vi "Read Configured Load DeviceIDs.vi"(8 "error in":errorcluster, 11 "EMS Generic in":refnum<class "EMS Generic.lvclass">) -> (0 "error out":errorcluster, 2 "Load DeviceIDs":T1[](array[typedef]), 3 "EMS Generic out":refnum<class "EMS Generic.lvclass">)   [LabVIEW 2018, in "EMS Generic Actor.lvlib" / "EMS Generic.lvclass"]
uses:
  EMS Generic.lvclass
  <vilib>/ORNL/CSEISMIC DDS/CSEISMIC DDS Base/Data Types/Controls/DeviceID.ctl
  EMS Generic.lvclass/EMS Generic.ctl
  <vilib>/ORNL/CSEISMIC DDS/CSEISMIC DDS Base/Data Types/Controls/DeviceClass Selector.ctl
  <vilib>/ORNL/CSEISMIC DDS/CSEISMIC DDS Base/CSEISMIC DDS.lvclass
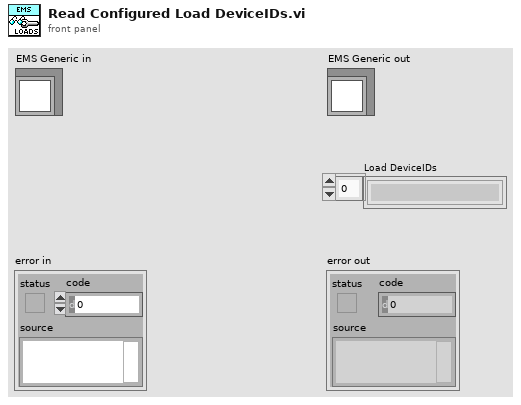
[diagram p1: front panel]
types:
  T1 = typedef "CSEISMIC DDS.lvlib/CSEISMIC DDS.lvclass/DeviceID.ctl" = string
  T2 = typedef "EMS Generic Actor.lvlib/EMS Generic.lvclass/Global Configuration.ctl" = cluster{"Microgrid ID":u8, "VF Device ID":T1, "Ongrid VF Priority":T1[], "Offgrid VF Priority":T1[], "AutoSwap Offgrid VF":u32, "AutoSwap Offgrid VF Delay (sec)":dbl, "AutoSwap Resynch VF":u32, "PCC Device ID":T1, "Device ID Array":T1[], "Nominal Voltage":dbl, "Nominal Frequency":dbl, "Resynch Timeout (sec)":dbl, "Island VF Activate Timeout (sec)":dbl, "Island PCC Target Power (kW)":dbl, "Island PCC Target Power Timeout (sec)":dbl, "Island Grid Settle Time (sec)":dbl, "Island PCC Failure Timeout (sec)":dbl, "Activation Devices Present Timeout (sec)":dbl, "Activation Devices Activated Timeout (sec)":dbl, "Blackstart VF GenMode Wait (sec)":dbl, "Blackstart VF DERCtrl Wait (sec)":dbl, "Blackstart Success Wait (sec)":dbl, "OnGrid Optimization Delay (sec)":dbl, "OffGrid Optimization Delay (sec)":dbl, "Resynch Frequency (Hz)":dbl, "Optimization Path":string}
  T3 = typedef "CSEISMIC DDS.lvlib/CSEISMIC DDS.lvclass/DeviceClass Selector.ctl" = u16
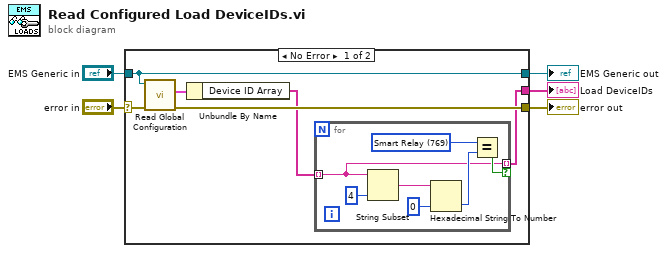
[diagram p0: block diagram]
diagram:
  n1 = case shown="No Error" "error in" {
    selector: "error in" -> [w10 w20]
    tunnel: [w8 w20] -> w4
    tunnel: [w11 w19] -> w2
    tunnel: "EMS Generic in" -> [w11 w19]
    tunnel: [w7 _] -> w1
    frame No Error {
      n2 = call "Read Global Configuration.vi"("error in"=w10, "EMS Generic in"=w11) -> ("error out"=w8:errorcluster, "Global Configuration"=w9:T2)  [unwired: 7 in, 1 out]
      n3 = Unbundle By Name(w9) -> ("Device ID Array"=w6:T1[])
      n4 = for {
        tunnel: [w12] -> w7 mode=indexing if=w13
        tunnel: w6 -> [w12] mode=indexing
        w16 = T3 769 items=["Invalid"=0, "IED"=256, "DER"=512, "Relay"=768, "Meter"=1024, "Load"=1280, "Forecast"=1536, "Price"=1792, "Energy Storage"=513, "PV"=514, "Generator"=515, "Smart Relay"=769, "PCC"=770, "Smart Meter"=1025, "PMU"=1026, "HVAC"=1281] ("DeviceClass")
        n5 = String Subset(string=w12, length (rest)=4 ("length (rest)")) -> (substring=w14:T1)  [unwired: 1 in]
        n6 = Hexadecimal String To Number(string=w14, default (0uL)=u16 0 ("default (0 U32)")) -> (number=w15:u16)  [unwired: 1 in, 1 out]
        n7 = Equal?(x=w16, y=w15) -> (x = y?=w13:bool)
      }
    }
    frame Error {
    }
  }
  "error out" <- w4
  "EMS Generic out" <- w2
  "Load DeviceIDs" <- w1
